vi "EqAreaAnnuli.vi"() -> ()   [LabVIEW 2022 SP3]
uses:
  <vilib>/Analysis/7linalg.llb/Solve Linear Equations (single right hand).vi
  <vilib>/Analysis/baseanly.llb/Solve Linear Equations By Cholesky.vi
  <vilib>/Analysis/baseanly.llb/Real Matrix to Compact Array.vi
  <vilib>/Analysis/baseanly.llb/Real Compact Tri-Matrix Linear Eqs.vi
  <vilib>/Analysis/7linalg.llb/Solve Linear Eqs (General).vi
  <vilib>/Analysis/7linalg.llb/Solve Linear Eqs (Gen, single right hand).vi
  <vilib>/Analysis/NI_AALPro.lvlib
panel:
  out "Solution Vector":dbl[](array[numeric]) format="%.2f"
  in  "Outer Rad":dbl format="%.2f"
  in  "Inner Rad":dbl format="%.2f"
  in  "Number of Rings":i16
  # "Solution includes inner and outer radious also"
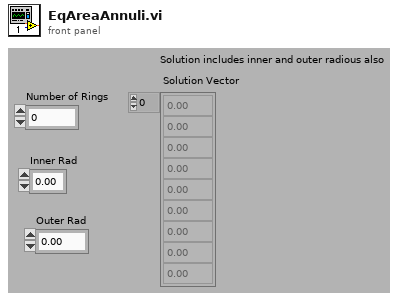
[diagram p1: front panel]
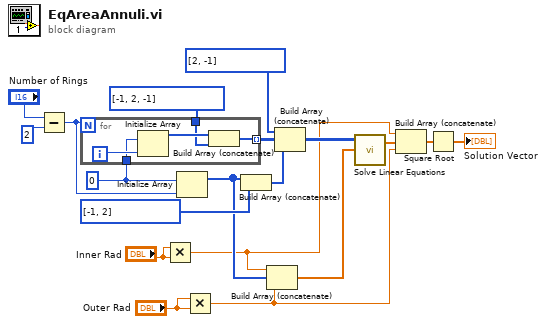
[diagram p0: block diagram]
diagram:
  w14 = 0
  n1 = Subtract(x="Number of Rings", y=2) -> (x-y=w13:i32)
  n2 = for {
    N: w13 -> [_]
    tunnel: i32[] [-1, 2, -1] -> [w22]
    tunnel: [w21] -> w16 mode=indexing
    tunnel: w14 -> [w20]
    i -> [w24]
    n3 = Initialize Array(w20, w24) -> (w23:i32[])
    n4 = Build Array (concatenate)(w23, w22) -> (w21:i32[])
  }
  n5 = Multiply(x="Inner Rad", y="Inner Rad") -> (x*y=w2:dbl)
  n6 = Initialize Array(w14, w13) -> (w9:i32[])
  n7 = Multiply(x="Outer Rad", y="Outer Rad") -> (x*y=w3:dbl)
  n8 = Build Array (concatenate)(w9, i32[] [-1, 2]) -> (w11:i32[])
  n9 = Build Array (concatenate)(w2, w9, w3) -> (w6:dbl[])
  n10 = Build Array (concatenate)(i32[] [2, -1], w16, w11) -> (w10:i32[][])
  n11 = call-poly <vilib>:"Solve Linear Equations.vi"("Known Vector"=w6, "Input Matrix"=w10) -> ("Solution Vector"=w4:dbl[])  [unwired: 1 in, 1 out]
  n12 = Build Array (concatenate)(w2, w4, w3) -> (w1:dbl[])
  n13 = Square Root(x=w1) -> (sqrt(x)=→"Solution Vector":dbl[])
